vi "ConvertSecondToStrTime.vi"(10 "type":enum16{"HHMMSS", "HH:MM:SS.S"}(ring), 11 "Second":dbl) -> (3 "time string":string)   [LabVIEW 2018, in "Library-DataConvert.lvlib"]
uses:
  Library-DataConvert.lvlib
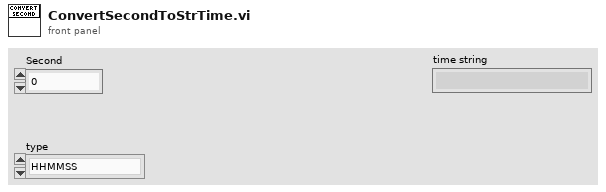
[diagram p1: front panel]
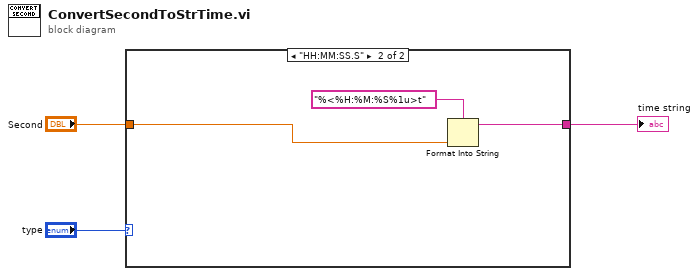
[diagram p0: block diagram]
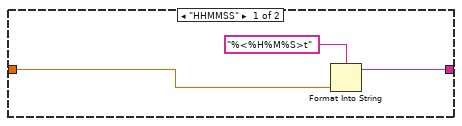
[diagram p2: hidden frame]
diagram:
  n1 = case shown="\"HH:MM:SS.S\"" "type" {
    tunnel: "Second" -> [w5 w8]
    tunnel: [w4 w7] -> w2
    frame "HHMMSS" {
      n2 = Format Into String(format string="%<%H%M%S>t" ("시간 포맷 문자열 (%c)"), w5) -> (resulting string=w4:string)  [unwired: 2 in, 1 out]
    }
    frame "HH:MM:SS.S" {
      n3 = Format Into String(format string="%<%H:%M:%S%1u>t" ("시간 포맷 문자열 (%c)"), w8) -> (resulting string=w7:string)  [unwired: 2 in, 1 out]
    }
  }
  "time string" <- w2
